vi "Distribute Controls Evenly.vi"(6 "space(6)":u32=6, 8 "error in (no error)":errorcluster, 11 "Controls":refnum<vi>[](array[refnum])) -> (0 "error out":errorcluster)   [LabVIEW 2017, in "csm-ui-support.lvlib"]
uses:
  csm-ui-support.lvlib
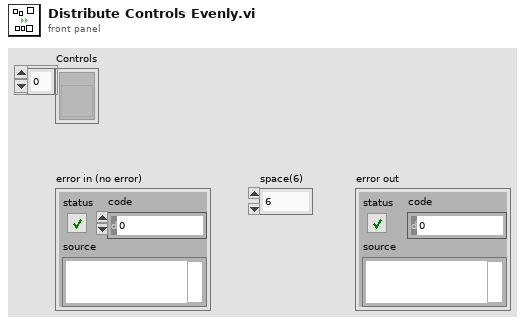
[diagram p1: front panel]
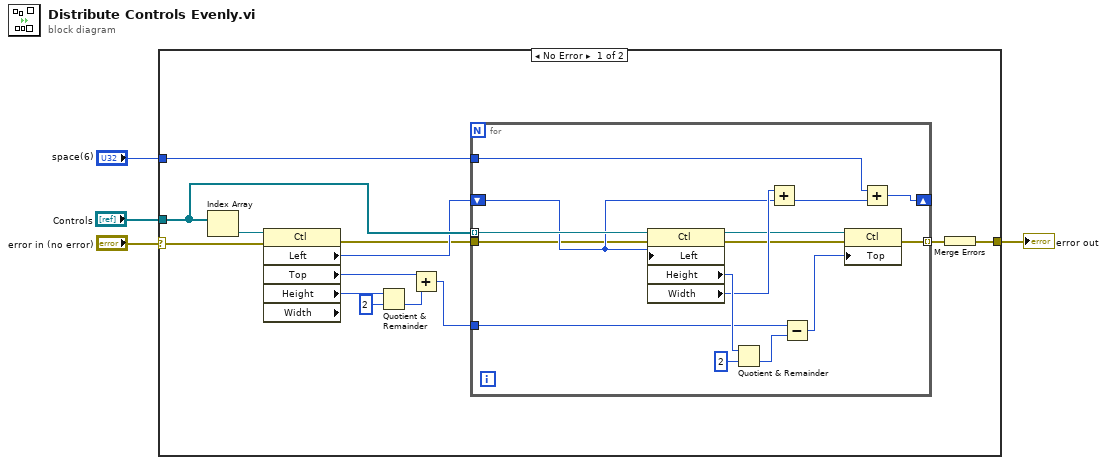
[diagram p0: block diagram]
diagram:
  n1 = case shown="No Error" "error in (no error)" {
    selector: "error in (no error)" -> [w8 w33]
    tunnel: "Controls" -> [w13 _]
    tunnel: [w6 w33] -> w4
    tunnel: "space(6)" -> [w5 _]
    frame No Error {
      n2 = Index Array(array=w13) -> (element=w14:refnum<vi>)  [unwired: 1 in]
      n3 = property class="Ctl" props=["Left", "Top", "Height", "Width"](reference=w14, error in=w8) -> (error out=w9:errorcluster, "Left"=w10:i32, "Top"=w17:i32, "Height"=w12:u32)  [unwired: 2 out]
      n4 = Quotient & Remainder(x=w12, y=u32 2) -> (floor(x/y)=w15:u32)  [unwired: 1 out]
      n5 = Add(x=w17, y=w15) -> (x+y=w11:u32)
      n6 = for {
        tunnel: w13 -> [w31] mode=indexing
        shift-right: [w32] -> _
        shift-left: w10 -> [w22]
        tunnel: w11 -> [w28]
        tunnel: w9 -> [w21]
        tunnel: [w19] -> w7 mode=indexing
        tunnel: w5 -> [w18]
        n7 = property class="Ctl"(reference=w31, error in=w21, "Left"=w22) -> (reference out=w23:refnum<vi>, error out=w20:errorcluster, "Height"=w29:u32, "Width"=w24:u32)
        n8 = Quotient & Remainder(x=w29, y=u32 2) -> (floor(x/y)=w27:u32)  [unwired: 1 out]
        n9 = Add(x=w24, y=w22) -> (x+y=w25:u32)
        n10 = Subtract(x=w28, y=w27) -> (x-y=w26:u32)
        n11 = property class="Ctl"(reference=w23, error in=w20, "Top"=w26) -> (error out=w19:errorcluster)  [unwired: 1 out]
        n12 = Add(x=w18, y=w25) -> (x+y=w32:u32)
      }
      n13 = Merge Errors(w7) -> (w6:errorcluster)
    }
    frame Error {
    }
  }
  "error out" <- w4
